vi "0mqCommv1.vi"(10 "intercomm configuration":T1) -> (0 "last error":errorcluster)   [LabVIEW 2018]
uses:
  Custom/S4msg.ctl
  <vilib>/addons/zeromq/socket_type.ctl
  <vilib>/addons/zeromq/zeromq.lvlib
  <vilib>/addons/zeromq/zmq_context.lvclass
  <vilib>/addons/zeromq/zmq_socket.lvclass
panel:
  out "last tick":u32
  in  "endpoint":string="localhost"
  out "S4ICS_status":string caption="Status received from S4ICS"
  out "S4ICS_command":string caption="Command sent to S4ICS"
  in  "Stop Client":bool
  # "S4ICS 0mqCOMM"
  # "COMMUNICATION CHANNEL"
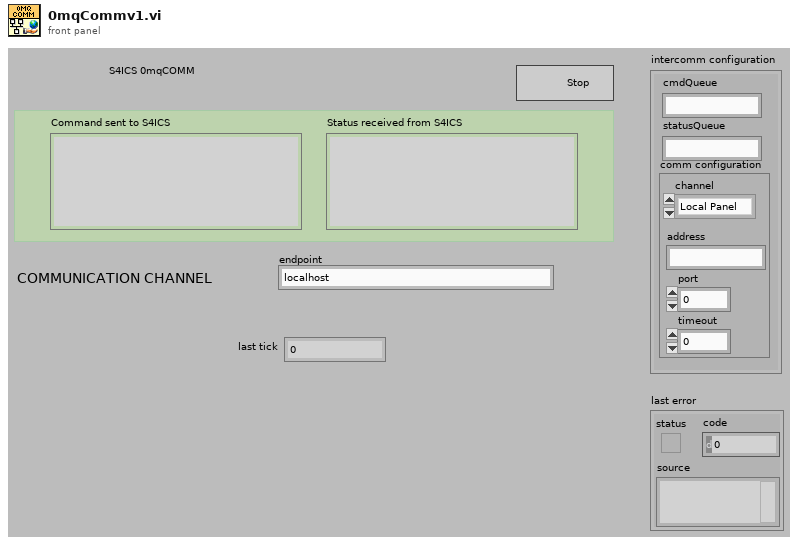
[diagram p1: front panel]
types:
  T1 = cluster{"S4commandQueueName":string, "S4statusQueueName":string, "comm configuration":cluster{"channel":enum32{"Local Panel", "Inner TCP/IP", "Outer TCP/IP", "MQTT", "ZeroMQ"}, "address":string, "port":u16, "timeout":i32}}
  T2 = typedef "zeromq.lvlib/socket_type.ctl" = enum8{"ZMQ_PAIR", "ZMQ_PUB", "ZMQ_SUB", "ZMQ_REQ", "ZMQ_REP", "ZMQ_DEALER", "ZMQ_ROUTER", "ZMQ_PULL", "ZMQ_PUSH", "ZMQ_XPUB", "ZMQ_XSUB", "ZMQ_STREAM", "ZMQ_SERVER", "ZMQ_CLIENT", "ZMQ_RADIO", "ZMQ_DISH", "ZMQ_GATHER", "ZMQ_SCATTER", "ZMQ_DGRAM"}
  T3 = typedef "S4msg.ctl" = cluster{"msg topic":string, "msg data":variant}
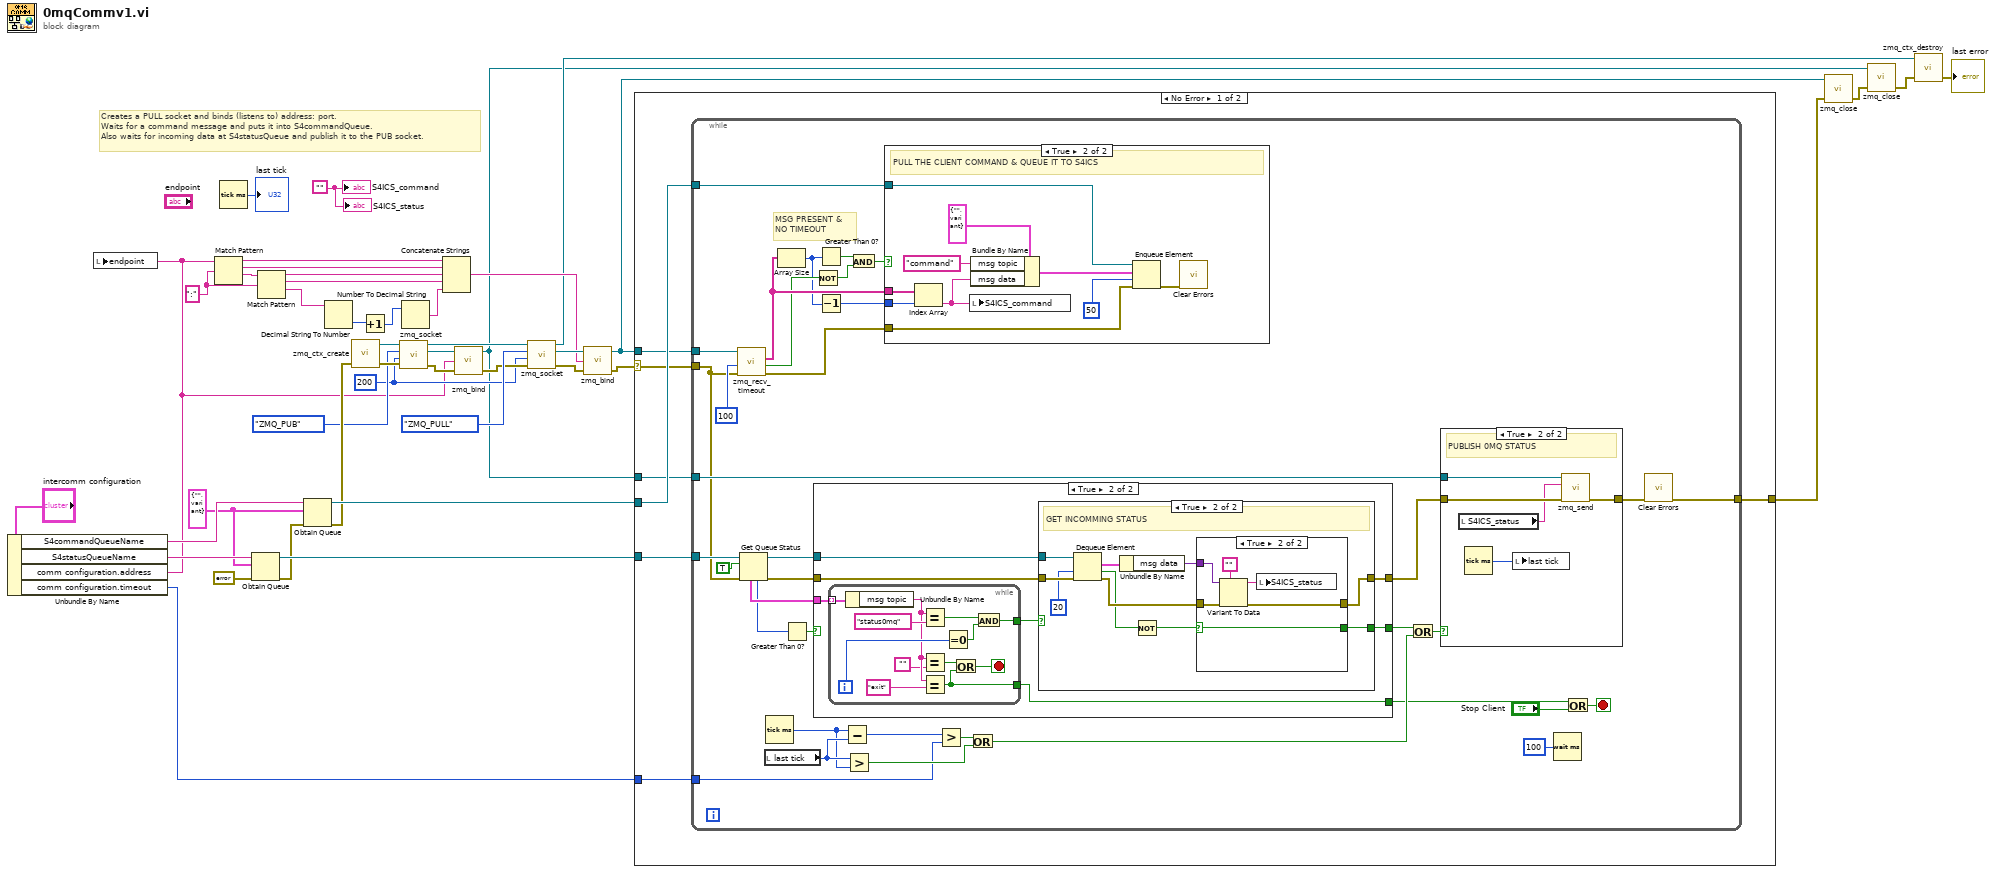
[diagram p0: block diagram]
diagram:
  w18 = 200 ("linger (ms)")
  w5 = ":" ("regular expression")
  w35 = T3 {"msg topic"="", "msg data"=variant} ("S4msg")
  w43 = ""
  # "Creates a PULL socket and binds (listens to) address: port. \nWaits for a command message and puts it into S4commandQueue.  \nAlso waits for incoming data at S4statusQueue and publish it to the PUB socket."
  n1 = Unbundle By Name("intercomm configuration") -> ("S4commandQueueName"=w41:string, "S4statusQueueName"=w42:string, "comm configuration.address"=w7:string, "comm configuration.timeout"=w8:i32)
  n2 = local write "endpoint"(w7) -> ()
  n3 = Match Pattern(string=w7, regular expression=w5) -> (before substring=w22:string, match substring=w21:string, after substring=w6:string)  [unwired: 1 in, 1 out]
  n4 = Tick Count (ms)() -> (millisecond timer value=→"last tick":u32)
  n5 = Obtain Queue(name (unnamed)=w42, element data type=w35, error in (no error)=errorcluster {"status"=FALSE, "code"=0, "source"=""}) -> (queue out=w39:refnum<queue>, error out=w36:errorcluster)  [unwired: 2 in, 1 out]
  n6 = Match Pattern(string=w6, regular expression=w5) -> (before substring=w3:string, match substring=w2:string, after substring=w1:string)  [unwired: 1 in, 1 out]
  n7 = Obtain Queue(name (unnamed)=w41, element data type=w35, error in (no error)=w36) -> (queue out=w40:refnum<queue>, error out=w38:errorcluster)  [unwired: 2 in, 1 out]
  n8 = Decimal String To Number(string=w1) -> (number=w24:i32)  [unwired: 2 in, 1 out]
  n9 = call <vilib>:"zmq_ctx_create.vi"("error in"=w38) -> ("error out"=w33:errorcluster, "context out"=w27:refnum<class "zmq_context.lvclass">)  [unwired: 3 in]
  n10 = Increment(x=w24) -> (x+1=w23:i32)
  n11 = call <vilib>:"zmq_socket.vi"("error in"=w33, "linger (ms)"=w18, "socket type"=socket_type."ZMQ_PUB", "context in"=w27) -> ("error out"=w34:errorcluster, "socket out"=w31:refnum<class "zmq_socket.lvclass">, "context out"=w20:refnum<class "zmq_context.lvclass">)  [unwired: 1 in]
  n12 = Number To Decimal String(number=w23) -> (decimal integer string=w4:string)  [unwired: 1 in]
  n13 = Concatenate Strings(w22, w21, w3, w2, w4) -> (w17:string)
  n14 = call <vilib>:"zmq_bind.vi"("error in"=w34, "endpoint"=w7, "socket in"=w31) -> ("error out"=w19:errorcluster, "socket out"=w10:refnum<class "zmq_socket.lvclass">)  [unwired: 1 in]
  n15 = call <vilib>:"zmq_socket.vi"("error in"=w19, "linger (ms)"=w18, "socket type"=socket_type."ZMQ_PULL", "context in"=w20) -> ("error out"=w30:errorcluster, "socket out"=w28:refnum<class "zmq_socket.lvclass">, "context out"=w11:refnum<class "zmq_context.lvclass">)  [unwired: 1 in]
  n16 = call <vilib>:"zmq_bind.vi"("error in"=w30, "endpoint"=w17, "socket in"=w28) -> ("error out"=w16:errorcluster, "socket out"=w9:refnum<class "zmq_socket.lvclass">)  [unwired: 1 in]
  n17 = case shown="No Error" w16 {
    selector: w16 -> [w46 w144]
    tunnel: w40 -> [w50 _]
    tunnel: w39 -> [w49 _]
    tunnel: w9 -> [w48 _]
    tunnel: w10 -> [w47 _]
    tunnel: [w45 w144] -> w14
    tunnel: w8 -> [w44 _]
    frame No Error {
      n18 = while {
        tunnel: [w62] -> w45
        tunnel: w50 -> [w67]
        tunnel: w49 -> [w86]
        tunnel: w48 -> [w74]
        tunnel: w47 -> [w78]
        tunnel: w46 -> [w63]
        tunnel: w44 -> [w58]
        stop <- w61 stop-if-true
        # "MSG PRESENT &\nNO TIMEOUT"
        n19 = call <vilib>:"zmq_recv_timeout.vi"("error in"=w63, "timeout (ms)"=u32 100, "socket in"=w74) -> ("error out"=w66:errorcluster, "timeout?"=w69:bool, "parts"=w72:string[])  [unwired: 1 in, 1 out]
        n20 = Get Queue Status(queue=w86, return elements? (F)=TRUE, error in (no error)=w63) -> (queue out=w56:refnum<queue>, error out=w55:errorcluster, # elements in queue=w52:i32, elements=w54:T3[])  [unwired: 4 out]
        n21 = local read "last tick"() -> (w84:u32)
        n22 = Tick Count (ms)() -> (millisecond timer value=w83:u32)
        n23 = Array Size(array=w72) -> (size(s)=w65:i32)
        n24 = Greater Than 0?(x=w52) -> (x > 0?=w53:bool)
        n25 = Not(x=w69) -> (.not. x?=w70:bool)
        n26 = case shown="True" w53 {
          selector: w53 -> [w87 _]
          tunnel: [w88 w95] -> w77
          tunnel: [w87 w93] -> w75
          tunnel: [w87 w92] -> w59
          tunnel: w56 -> [_ w91]
          tunnel: w55 -> [w88 w90]
          tunnel: w54 -> [_ w89]
          frame False {
          }
          frame True {
            n27 = while {
              tunnel: [w101] -> w94
              tunnel: [w97] -> w92
              tunnel: w89 -> [w105] mode=indexing
              i -> [w104]
              stop <- w96 stop-if-true
              n28 = Unbundle By Name(w105) -> ("msg topic"=w100:string)
              n29 = Equal?(x=w100, y="status0mq" ("msg topic")) -> (x = y?=w103:bool)
              n30 = Equal?(x=w100, y="") -> (x = y?=w98:bool)
              n31 = Equal?(x=w100, y="exit" ("msg topic")) -> (x = y?=w97:bool)
              n32 = Equal To 0?(x=w104) -> (x = 0?=w102:bool)
              n33 = Or(x=w98, y=w97) -> (x .or. y?=w96:bool)
              n34 = And(x=w103, y=w102) -> (x .and. y?=w101:bool)
            }
            n35 = case shown="True" w94 {
              selector: w94 -> [w108 _]
              tunnel: w90 -> [w109 w119]
              tunnel: w91 -> [_ w118]
              tunnel: [w109 w114] -> w95
              tunnel: [w108 w110] -> w93
              frame False {
              }
              frame True {
                # "GET INCOMMING STATUS"
                n36 = Dequeue Element(queue=w118, timeout in ms (-1)=20, error in (no error)=w119) -> (element=w117:T3, timed out?=w112:bool, error out=w115:errorcluster)  [unwired: 1 out]
                n37 = Unbundle By Name(w117) -> ("msg data"=w116:variant)
                n38 = Not(x=w112) -> (.not. x?=w111:bool)
                n39 = case shown="True" w111 {
                  selector: w111 -> [w121 w122]
                  tunnel: w116 -> [_ w127]
                  tunnel: w115 -> [w120 w126]
                  tunnel: [w120 w125] -> w114
                  tunnel: [w121 w122] -> w110
                  frame False {
                  }
                  frame True {
                    n40 = Variant To Data(error in=w126, type="", Variant=w127) -> (data=w123:string, error out=w125:errorcluster)
                    n41 = local write "S4ICS_status"(w123) -> ()
                  }
                }
              }
            }
          }
        }
        n42 = Greater Than 0?(x=w65) -> (x > 0?=w71:bool)
        n43 = Decrement(x=w65) -> (x-1=w64:i32)
        n44 = Subtract(x=w83, y=w84) -> (x-y=w85:u32)
        n45 = Greater?(x=w84, y=w83) -> (0:w81:bool)
        n46 = And(x=w71, y=w70) -> (x .and. y?=w68:bool)
        n47 = case shown="True" w68 {
          tunnel: w72 -> [_ w136]
          tunnel: w67 -> [_ w131]
          tunnel: w66 -> [_ w130]
          tunnel: w64 -> [_ w129]
          frame False {
          }
          frame True {
            # "PULL THE CLIENT COMMAND & QUEUE IT TO S4ICS"
            n48 = Index Array(array=w136, index=w129) -> (element=w133:string)
            n49 = local write "S4ICS_command"(w133) -> ()
            n50 = Bundle By Name(cluster=T3 {"msg topic"="", "msg data"=variant} ("S4msg"), "msg topic"="command", "msg data"=w133) -> (w132:T3)
            n51 = Enqueue Element(queue=w131, element=w132, timeout in ms (-1)=50, error in (no error)=w130) -> (error out=w128:errorcluster)  [unwired: 2 out]
            n52 = call <vilib>:"Clear Errors.vi"("error in (no error)"=w128) -> ()  [unwired: 5 in, 2 out]
          }
        }
        n53 = Greater?(x=w85, y=w58) -> (0:w82:bool)
        n54 = Or(x=w82, y=w81) -> (x .or. y?=w80:bool)
        n55 = Or(x=w75, y=w80) -> (x .or. y?=w79:bool)
        n56 = case shown="True" w79 {
          tunnel: [w138 w139] -> w76
          tunnel: w78 -> [_ w143]
          tunnel: w77 -> [w138 w142]
          frame False {
          }
          frame True {
            # "PUBLISH 0MQ STATUS"
            n57 = local read "S4ICS_status"() -> (w141:string)
            n58 = Tick Count (ms)() -> (millisecond timer value=w140:u32)
            n59 = local write "last tick"(w140) -> ()
            n60 = call <vilib>:"zmq_send.vi"("error in"=w142, "data"=w141, "socket in"=w143) -> ("error out"=w139:errorcluster)  [unwired: 4 in, 1 out]
          }
        }
        n61 = Wait (ms)(milliseconds to wait=u32 100) -> ()  [unwired: 1 out]
        n62 = Or(x=w59, y="Stop Client") -> (x .or. y?=w61:bool)
        n63 = call <vilib>:"Clear Errors.vi"("error in (no error)"=w76) -> ("error out"=w62:errorcluster)  [unwired: 5 in, 1 out]
      }
    }
    frame Error {
    }
  }
  n64 = call <vilib>:"zmq_close.vi"("error in"=w14, "socket"=w9) -> ("error out"=w13:errorcluster)  [unwired: 3 in]
  n65 = call <vilib>:"zmq_close.vi"("error in"=w13, "socket"=w10) -> ("error out"=w15:errorcluster)  [unwired: 3 in]
  n66 = call <vilib>:"zmq_ctx_destroy.vi"("error in"=w15, "context in"=w11) -> ("error out"=→"last error":errorcluster)  [unwired: 3 in]
  "S4ICS_command" <- w43
  "S4ICS_status" <- w43
